vi "sum of num using inc,shift reg,for loop.vi"() -> ()   [LabVIEW 2025]
panel:
  out "sum of number":dbl
  in  "enter a num":dbl
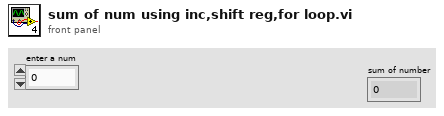
[diagram p1: front panel]
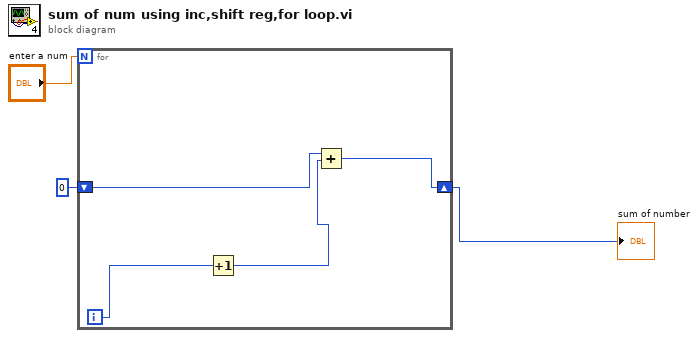
[diagram p0: block diagram]
diagram:
  n1 = for {
    N: "enter a num" -> [_]
    shift-right: [w5] -> w2
    shift-left: 0 -> [w4]
    i -> [w7]
    n2 = Increment(x=w7) -> (x+1=w6:i32)
    n3 = Add(x=w4, y=w6) -> (x+y=w5:i32)
  }
  "sum of number" <- w2
